vi "Path Test.vi"   [LabVIEW 2020]
uses:
  build/ppl/neg-pkg.lvlibp
  MGI Console/Source/Console/Console.lvclass
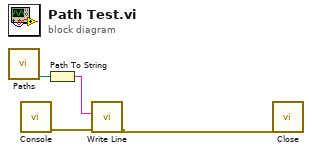
[diagram p0: block diagram]
diagram:
  n1 = call "Paths.vi"() -> ("ppl Path"=w2:path)  [unwired: 8 in, 3 out]
  n2 = call "Console.vi"() -> ("error out"=w4:errorcluster)  [unwired: 11 in]
  n3 = Path To String(path=w2) -> (string=w3:string)
  n4 = call "Write Line.vi"("error in (no error)"=w4, "Line"=w3) -> ("error out"=w1:errorcluster)  [unwired: 9 in]
  n5 = call "Close.vi"("error in (no error)"=w1) -> ()  [unwired: 10 in, 1 out]
